vi "Teleop.vi"(8 "error in (no error)":errorcluster, 9 "Joystick Data":T2, 10 "Robot Data In":T1, 11 "Outlaw in":refnum<class "Outlaw.lvclass">) -> (0 "error out":errorcluster, 2 "Robot Data Out":T1, 3 "Outlaw out":refnum<class "Outlaw.lvclass">)   [LabVIEW 2019, in "Robot.lvlib" / "Outlaw.lvclass"]
uses:
  Outlaw.lvclass
  Robot.lvclass
  Vision/Vision.lvclass
  Elevator/Elevator.lvclass
  Pnematics control/Solenoids/Solenoids.lvclass
  Cargo/Cargo.lvclass
  Pnematics control/Pneumatics.lvclass
  Hatch/Hatch.lvclass
  DriveOld/Drive.lvclass
  Joysticks/Controls/JoystickData.ctl
  Joysticks/Joysticks.lvclass
  Drive/Tank Drive/Tank Drive.lvclass
  TypeDefs/RobotObjects.ctl
  Control Panel/Control Panel.lvclass
  Climber/Climber.lvclass
  Turret/Turret.lvclass
  PowerCellHandler/Power Cell Handler.lvclass
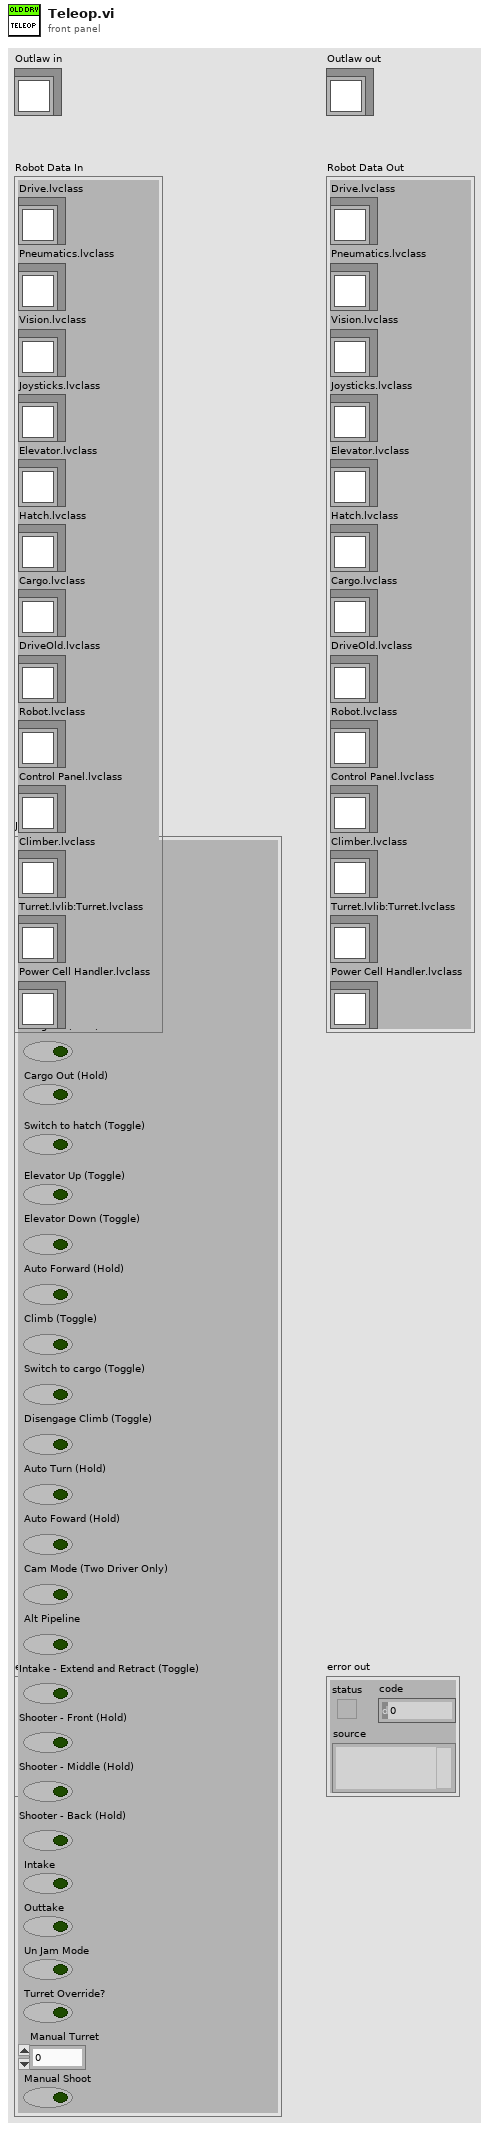
[diagram p1: front panel]
types:
  T1 = typedef "RobotObjects.ctl" = cluster{"Drive.lvclass":refnum<class "Tank Drive.lvclass">, "Pneumatics.lvclass":refnum<class "Pneumatics.lvclass">, "Vision.lvclass":refnum<class "Vision.lvclass">, "Joysticks.lvclass":refnum<class "Joysticks.lvclass">, "Elevator.lvclass":refnum<class "Elevator.lvclass">, "Hatch.lvclass":refnum<class "Hatch.lvclass">, "Cargo.lvclass":refnum<class "Cargo.lvclass">, "DriveOld.lvclass":refnum<class "Drive.lvclass">, "Robot.lvclass":refnum<class "Robot.lvclass">, "Control Panel.lvclass":refnum<class "Control Panel.lvclass">, "Climber.lvclass":refnum<class "Climber.lvclass">, "Turret.lvlib:Turret.lvclass":refnum<class "Turret.lvclass">, "Power Cell Handler.lvclass":refnum<class "Power Cell Handler.lvclass">}
  T2 = typedef "Joysticks.lvlib/Joysticks.lvclass/JoystickData.ctl" = cluster{"X Axis ":dbl, "Y Axis":dbl, "Drivetrain Shifter (Hold)":bool, "Beak (Toggle)":bool, "Cargo In (Hold)":bool, "Cargo Out (Hold)":bool, "Switch to hatch (Toggle)":bool, "Elevator Up (Toggle)":bool, "Elevator Down (Toggle)":bool, "Auto Forward (Hold)":bool, "Climb (Toggle)":bool, "Switch to cargo (Toggle)":bool, "Disengage Climb (Toggle)":bool, "Auto Turn (Hold)":bool, "Auto Foward (Hold)":bool, "Cam Mode (Two Driver Only)":bool, "Alt Pipeline":bool, "Intake - Extend and Retract (Toggle)":bool, "Shooter - Front (Hold)":bool, "Shooter - Middle (Hold)":bool, "Shooter - Back (Hold)":bool, "Intake":bool, "Outtake":bool, "Un Jam Mode":bool, "Turret Override?":bool, "Manual Turret":dbl, "Manual Shoot":bool}
  T3 = typedef "Pneumatics control.lvlib/Pneumatics.lvclass/Solenoids.ctl" = cluster{"Air Cooler":refnum<class "Solenoids.lvclass">, "ArmLock":refnum<class "Solenoids.lvclass">, "HatchArm":refnum<class "Solenoids.lvclass">, "HatchGrabber":refnum<class "Solenoids.lvclass">, "CPDeploy":refnum<class "Solenoids.lvclass">, "Power Cells Intake":refnum<class "Solenoids.lvclass">}
  T4 = typedef "Elevator.lvlib/Elevator.lvclass/Elevator Position.ctl" = enum16{"CS, Cargo Ship Cargo", "C0, Cargo Ground", "C1, LV1 Cargo", "C2, LV2 Cargo", "C3, LV3 Cargo", "H0, LV1 Hatch", "H1, LV2 Hatch", "H2, LV3 Hatch"}
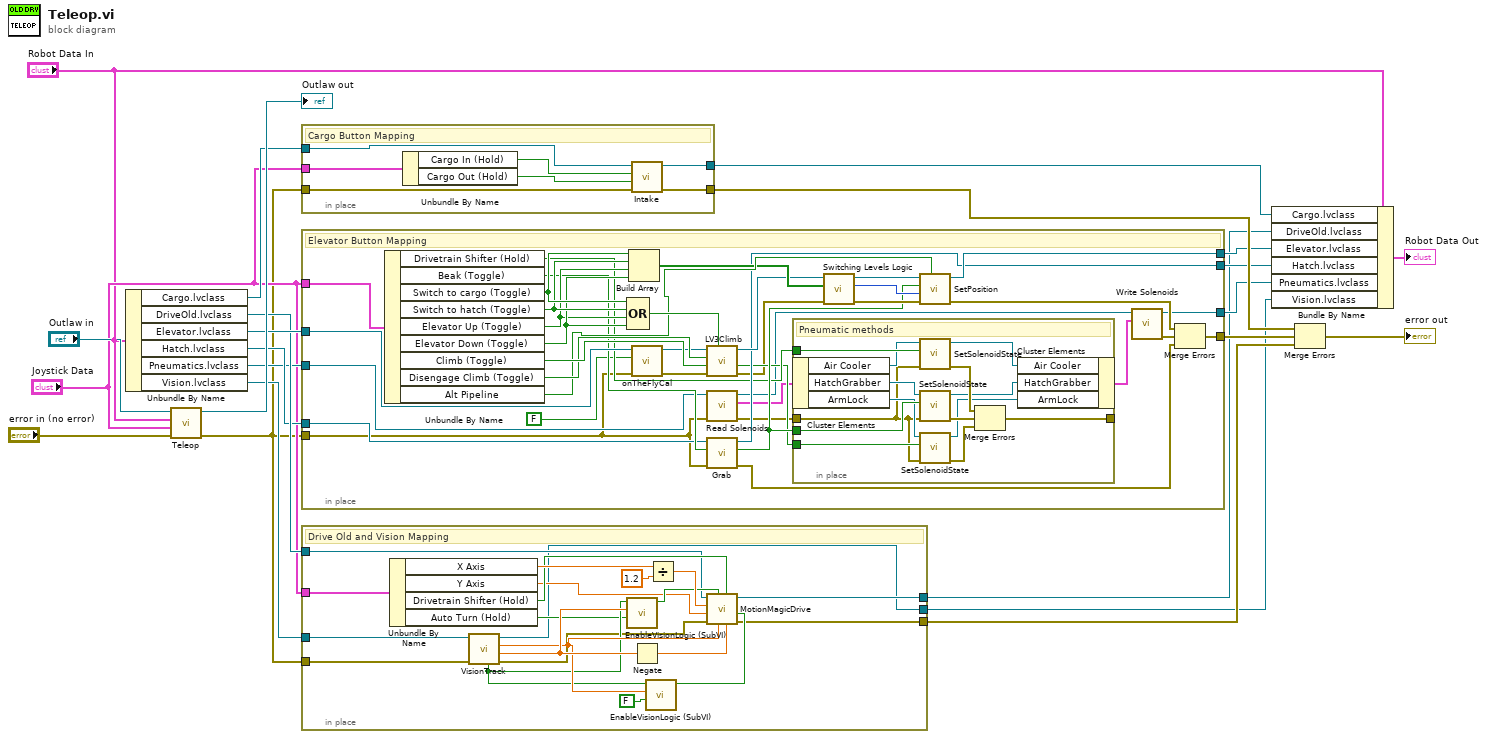
[diagram p0: block diagram]
diagram:
  n1 = Unbundle By Name("Robot Data In") -> ("Cargo.lvclass"=w14:refnum<class "Cargo.lvclass">, "DriveOld.lvclass"=w17:refnum<class "Drive.lvclass">, "Elevator.lvclass"=w18:refnum<class "Elevator.lvclass">, "Hatch.lvclass"=w15:refnum<class "Hatch.lvclass">, "Pneumatics.lvclass"=w13:refnum<class "Pneumatics.lvclass">, "Vision.lvclass"=w16:refnum<class "Vision.lvclass">)
  n2 = call-parent "Teleop.vi"("error in (no error)"="error in (no error)", "Joystick Data"="Joystick Data", "Robot Data In"="Robot Data In", "Robot in"="Outlaw in") -> ("error out"=w4:errorcluster, "Robot out"=→"Outlaw out":refnum<class "Outlaw.lvclass">)  [unwired: 5 in, 1 out]
  n3 = in-place {
    in-place-border: "Joystick Data" -> [w28]
    in-place-border: w14 -> [w27]
    in-place-border: [w26] -> w7
    in-place-border: w4 -> [w25]
    in-place-border: [w24] -> w12
    # "Cargo Button Mapping"
    n4 = Unbundle By Name(w28) -> ("Cargo In (Hold)"=w30:bool, "Cargo Out (Hold)"=w29:bool)
    n5 = call-dynamic "Intake.vi"("error in (no error)"=w25, "Out"=w29, "In"=w30, "Cargo in"=w27) -> ("error out"=w24:errorcluster, "Cargo out"=w26:refnum<class "Cargo.lvclass">)  [unwired: 6 in]
  }
  n6 = in-place {
    in-place-border: w4 -> [w43]
    in-place-border: [w37] -> w20
    in-place-border: "Joystick Data" -> [w54]
    in-place-border: w18 -> [w53]
    in-place-border: [w52] -> w8
    in-place-border: w15 -> [w50]
    in-place-border: [w49] -> w10
    in-place-border: w13 -> [w44]
    in-place-border: [w36] -> w11
    # "Elevator Button Mapping"
    n7 = Unbundle By Name(w54) -> ("Drivetrain Shifter (Hold)"=w47:bool, "Beak (Toggle)"=w51:bool, "Switch to cargo (Toggle)"=w62:bool, "Switch to hatch (Toggle)"=w61:bool, "Elevator Up (Toggle)"=w59:bool, "Elevator Down (Toggle)"=w60:bool, "Climb (Toggle)"=w66:bool, "Disengage Climb (Toggle)"=w65:bool, "Alt Pipeline"=w64:bool)
    n8 = Compound Arithmetic op=OR(w62, w61, w59, w60) -> (w67:bool)
    n9 = Build Array(w62, w61, w59, w60) -> (w63:bool[])
    n10 = call-dynamic "onTheFlyCal.vi"("error in (no error)"=w43, "calibrateElevator"=FALSE, "Elevator in"=w53) -> ("error out"=w45:errorcluster, "Elevator out"=w34:refnum<class "Elevator.lvclass">)  [unwired: 7 in]
    n11 = call-dynamic "LV3Climb.vi"("Deactivate?"=w67, "error in (no error)"=w45, "Activate?"=w66, "Redeploy?"=w65, "Elevator in"=w34) -> ("error out"=w33:errorcluster, "activate wrist lock"=w46:bool, "Elevator out"=w58:refnum<class "Elevator.lvclass">)  [unwired: 4 in]
    n12 = call-dynamic "Read Solenoids.vi"("error in (no error)"=w43, "Pneumatics in"=w44) -> ("error out"=w35:errorcluster, "Solenoids"=w41:T3, "Pneumatics out"=w42:refnum<class "Pneumatics.lvclass">)  [unwired: 7 in]
    n13 = call-dynamic "Grab.vi"("error in (no error)"=w43, "Grab Toggle?"=w51, "Hatch in"=w50) -> ("error out"=w32:errorcluster, "Solenoid On?"=w48:bool, "Hatch out"=w49:refnum<class "Hatch.lvclass">)  [unwired: 6 in]
    n14 = in-place {
      in-place-border: w47 -> [w80]
      in-place-border: w35 -> [w68]
      in-place-border: [w78] -> _
      in-place-border: w48 -> [w76]
      in-place-border: w46 -> [w69]
      # "Pneumatic methods"
      n15 = in-place-cluster #1(w41) -> ("Air Cooler"=w74:refnum<class "Solenoids.lvclass">, "HatchGrabber"=w73:refnum<class "Solenoids.lvclass">, "ArmLock"=w72:refnum<class "Solenoids.lvclass">)
      n16 = call-dynamic "SetSolenoidState.vi"("error in (no error)"=w68, "Solenoid On?"=w80, "Solenoids in"=w74) -> ("error out"=w79:errorcluster, "Solenoids out"=w81:refnum<class "Solenoids.lvclass">)  [unwired: 7 in]
      n17 = call-dynamic "SetSolenoidState.vi"("error in (no error)"=w68, "Solenoid On?"=w76, "Solenoids in"=w73) -> ("error out"=w77:errorcluster, "Solenoids out"=w71:refnum<class "Solenoids.lvclass">)  [unwired: 7 in]
      n18 = call-dynamic "SetSolenoidState.vi"("error in (no error)"=w68, "Solenoid On?"=w69, "Solenoids in"=w72) -> ("error out"=w75:errorcluster, "Solenoids out"=w70:refnum<class "Solenoids.lvclass">)  [unwired: 7 in]
      n19 = Merge Errors(w79, w77, w75) -> (w78:errorcluster)
      n20 = in-place-cluster #1("Air Cooler"=w81, "HatchGrabber"=w71, "ArmLock"=w70) -> (w40:T3)
    }
    n21 = call "Switching Levels Logic.vi"("error in (no error)"=w33, "buttons"=w63, "Elevator in"=w58) -> ("error out"=w57:errorcluster, "Cargo/Hatch"=w56:T4, "Elevator out"=w55:refnum<class "Elevator.lvclass">)  [unwired: 6 in]
    n22 = call-dynamic "SetPosition.vi"("AltPipe?"=w64, "error in (no error)"=w57, "Position"=w56, "Hatch Grabbed?"=w48, "Elevator in"=w55) -> ("error out"=w39:errorcluster, "Elevator out"=w52:refnum<class "Elevator.lvclass">)  [unwired: 5 in]
    n23 = call-dynamic "Write Solenoids.vi"("Solenoids"=w40, "Pneumatics in"=w42) -> ("error out"=w38:errorcluster, "Pneumatics out"=w36:refnum<class "Pneumatics.lvclass">)  [unwired: 8 in]
    n24 = Merge Errors(w39, w38, w32) -> (w37:errorcluster)
  }
  n25 = in-place {
    in-place-border: w4 -> [w88]
    in-place-border: "Joystick Data" -> [w89]
    in-place-border: [w86] -> w19
    in-place-border: w17 -> [w85]
    in-place-border: w16 -> [w84]
    in-place-border: [w83] -> w6
    in-place-border: [w82] -> w9
    # "Drive Old and Vision Mapping"
    n26 = Unbundle By Name(w89) -> ("X Axis"=w102:dbl, "Y Axis"=w90:dbl, "Drivetrain Shifter (Hold)"=w101:bool, "Auto Turn (Hold)"=w91:bool)
    n27 = call "VisionTrack.vi"("error in (no error)"=w88, "Vision in"=w84) -> ("error out"=w87:errorcluster, "VerticalOffset(degrees)"=w98:dbl, "HorizontalOffset(degrees)"=w96:dbl, "Vision out"=w82:refnum<class "Vision.lvclass">, "Target?"=w94:bool)  [unwired: 4 in, 1 out]
    n28 = call "EnableVisionLogic (SubVI).vi"("Activate?(hold)"=w91, "Offset(degrees)"=w98, "Target?"=w94) -> ("Enable?"=w97:bool)  [unwired: 8 in]
    n29 = Negate(x=w98) -> (-x=w93:dbl)
    n30 = call "EnableVisionLogic (SubVI).vi"("Activate?(hold)"=FALSE, "Offset(degrees)"=w96, "Target?"=w94) -> ("Enable?"=w95:bool)  [unwired: 8 in]
    n31 = Divide(x=w102, y=1.2) -> (x/y=w100:dbl)
    n32 = call-dynamic "MotionMagicDrive.vi"("Enable Vision Y"=w95, "X offset"=w93, "High gear?"=w101, "Y offset"=w96, "Enable Vision X"=w97, "error in (no error)"=w87, "Y Axis"=w90, "X Axis"=w100, "Drive in"=w85) -> ("error out"=w86:errorcluster, "Drive out"=w83:refnum<class "Drive.lvclass">)  [unwired: 1 in]
  }
  n33 = Bundle By Name(cluster="Robot Data In", "Cargo.lvclass"=w7, "DriveOld.lvclass"=w6, "Elevator.lvclass"=w8, "Hatch.lvclass"=w10, "Pneumatics.lvclass"=w11, "Vision.lvclass"=w9) -> (→"Robot Data Out":T1)
  n34 = Merge Errors(w12, w20, w19) -> (→"error out":errorcluster)
